vi "Load Localized Strings.vi"(7 "Mode":enum16{"Read", "Write"}(ring), 8 "error in (no error)":errorcluster, 11 "VI Refnum":refnum<vi>) -> (0 "error out":errorcluster, 3 "dup VI Refnum":refnum<vi>)   [LabVIEW 2020, in "Localization_Tools.lvlib"]
uses:
  Localization_Tools.lvlib
  LOC VI Tools Globals.vi
  <vilib>/Utility/config.llb/NI_LVConfig.lvlib
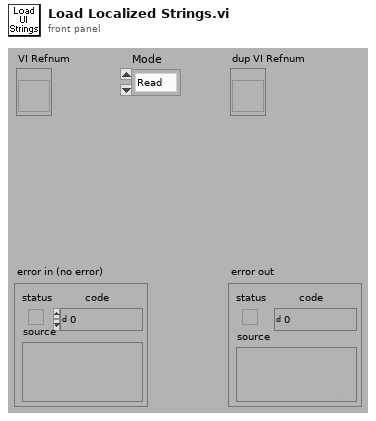
[diagram p1: front panel]
types:
  T1 = typedef "NI_LVConfig.lvlib/Config Data RefNum.ctl" = refnum<k1>
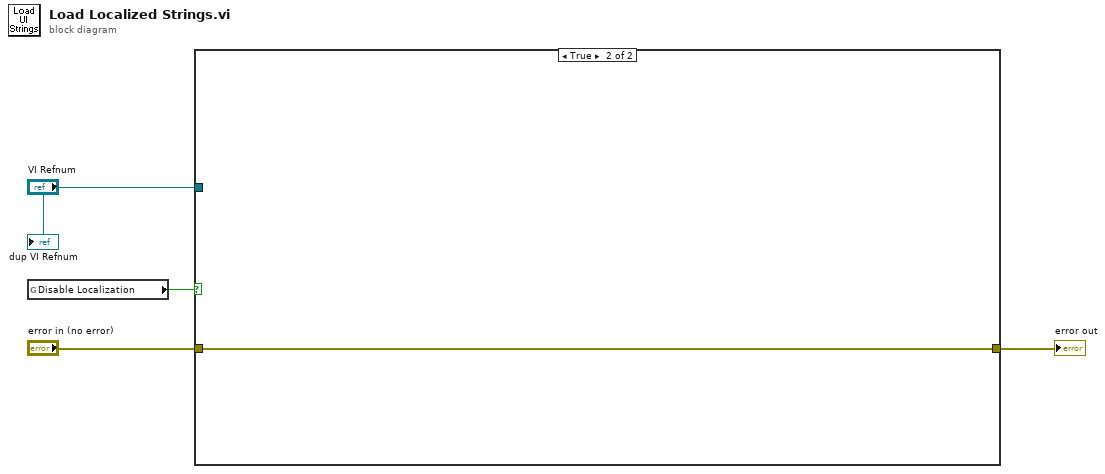
[diagram p0: block diagram]
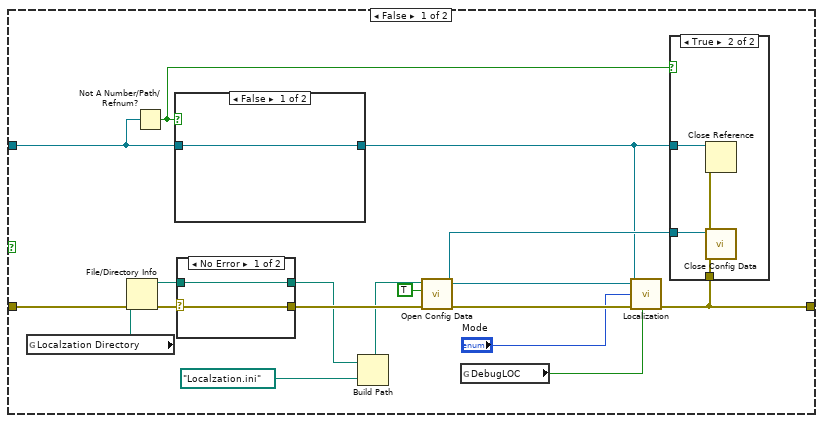
[diagram p2: hidden frame]
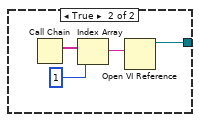
[diagram p4: hidden frame]
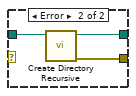
[diagram p5: hidden frame]
diagram:
  n1 = global read "LOC VI Tools Globals.vi" "Disable Localization"() -> (w1:bool)
  n2 = case shown="True" w1 {
    tunnel: [w21 w35] -> w3
    tunnel: "VI Refnum" -> [w20 _]
    tunnel: "error in (no error)" -> [w19 w35]
    frame False {
      n3 = global read "LOC VI Tools Globals.vi" "Localzation Directory"() -> (w5:path)
      n4 = File/Directory Info(path=w5, error in=w19) -> (path out=w18:path, error out=w16:errorcluster)  [unwired: 5 out]
      n5 = Not A Number/Path/Refnum?(number/path/refnum=w20) -> (NaN/Path/Refnum?=w8:bool)
      n6 = case shown="False" w8 {
        tunnel: w20 -> [w25 _]
        tunnel: [w25 w26] -> w7
        frame False {
        }
        frame True {
          n7 = Call Chain() -> (call chain=w27:string[])
          n8 = Index Array(array=w27, index=1) -> (element=w29:string)
          n9 = Open VI Reference(vi path=w29) -> (vi reference=w26:refnum<vi>)  [unwired: 5 in, 1 out]
        }
      }
      n10 = case shown="No Error" w16 {
        selector: w16 -> [w31 _]
        tunnel: w18 -> [w30 w34]
        tunnel: [w31 w33] -> w17
        tunnel: [w30 w32] -> w14
        frame No Error {
        }
        frame Error {
          n11 = call <vilib>:"Create Directory Recursive.vi"("directory"=w34) -> ("error out"=w33:errorcluster, "directory copy"=w32:path)  [unwired: 4 in, 1 out]
        }
      }
      n12 = Build Path(base path=w14, name or relative path=path "Localzation.ini") -> (appended path=w12:path)
      n13 = call <vilib>:"Open Config Data.vi"("error in (no error)"=w17, "create file if necessary (T)"=TRUE, "configuration file path"=w12) -> ("error out"=w15:errorcluster, "refnum"=w10:T1)  [unwired: 6 in, 1 out]
      n14 = global read "LOC VI Tools Globals.vi" "DebugLOC"() -> (w6:bool)
      n15 = call "Localization.vi"("OwningVIRefnum"=w7, "ConfigFileRefnum"=w10, "Mode"="Mode", "error in (no error)"=w15, "DebugLOC"=w6) -> ("error out"=w21:errorcluster)  [unwired: 3 in]
      n16 = case shown="True" w8 {
        tunnel: w7 -> [_ w24]
        tunnel: w21 -> [_ w23]
        tunnel: w10 -> [_ w22]
        frame False {
        }
        frame True {
          n17 = Close Reference(reference=w24, error in (no error)=w23) -> ()  [unwired: 1 out]
          n18 = call <vilib>:"Close Config Data.vi"("refnum"=w22) -> ()  [unwired: 9 in, 2 out]
        }
      }
    }
    frame True {
    }
  }
  "error out" <- w3
  "dup VI Refnum" <- "VI Refnum"
